vi "parseConstants.vi"(8 "error in (no error)":errorcluster, 10 "IDLString":string="module atcs {\n\tstruct LoopTime_ms {\n\t  string<32>\tprivate_revCode; //private\n\t  double\tprivate_sndStamp; //private\n\t  double\tprivate_rcvStamp; //private\n\t  long\t\tprivate_seqNum; //private\n\t  long\t\tprivate_origin; //private\n\t  long\t\tprivate_host; //private\n\t  double\tloopTime_ms;\n\t};\n\t#pragma keylist LoopTime_ms\n\tstruct Timestamp {\n\t  string<32>\tprivate_revCode; //private\n\t  double\tprivate_sndStamp; //private\n\t  double\tprivate_rcvStamp; //private\n\t  long\t\tprivate_seqNum; //private\n\t  long\t\tprivate_origin; //private\n\t  long\t\tprivate_host; //private\n\t  double\ttimestamp;\n\t};\n\t#pragma keylist Timestamp\n\tstruct command_Offset {\n\t  string<32>\tprivate_revCode; //private\n\t  double\tprivate_sndStamp; //private\n\t  double\tprivate_rcvStamp; //private\n\t  long\t\tprivate_seqNum; //private\n\t  long\t\tprivate_origin; //private\n\t  long\t\tprivate_host; //private\n\t  string<32>\tdevice;\n\t  string<32>\tproperty;\n\t  string<32>\taction;\n\t  string<32>\tvalue;\n\t  double\toffsetX;\n\t  double\toffsetY;\n\t};\n\t#pragma keylist command_Offset\n\tstruct command_SpectrographSetup {\n\t  string<32>\tprivate_revCode; //private\n\t  double\tprivate_sndStamp; //private\n\t  double\tprivate_rcvStamp; //private\n\t  long\t\tprivate_seqNum; //private\n\t  long\t\tprivate_origin; //private\n\t  long\t\tprivate_host; //private\n\t  string<32>\tdevice;\n\t  string<32>\tproperty;\n\t  string<32>\taction;\n\t  string<32>\tvalue;\n\t  long\tgrating;\n\t  long\tfilter;\n\t  double\tstagePosition;\n\t};\n\t#pragma keylist command_SpectrographSetup\n\tstruct command_Target {\n\t  string<32>\tprivate_revCode; //private\n\t  double\tprivate_sndStamp; //private\n\t  double\tprivate_rcvStamp; //private\n\t  long\t\tprivate_seqNum; //private\n\t  long\t\tprivate_origin; //private\n\t  long\t\tprivate_host; //private\n\t  string<32>\tdevice;\n\t  string<32>\tproperty;\n\t  string<32>\taction;\n\t  string<32>\tvalue;\n\t  long\ttargetId;\n\t  double\tra;\n\t  double\tdecl;\n\t  double\tskyPositionAngle;\n\t  long\tnumOfExposures;\n\t  double\texposureTime;\n\t};\n\t#pragma keylist command_Target\n\tstruct command_disable {\n\t  string<32>\tprivate_revCode; //private\n\t  double\tprivate_sndStamp; //private\n\t  double\tprivate_rcvStamp; //private\n\t  long\t\tprivate_seqNum; //private\n\t  long\t\tprivate_origin; //private\n\t  long\t\tprivate_host; //private\n\t  string<32>\tdevice;\n\t  string<32>\tproperty;\n\t  string<32>\taction;\n\t  string<32>\tvalue;\n\t  boolean\tdisable;\n\t};\n\t#pragma keylist command_disable\n\tstruct command_enable {\n\t  string<32>\tprivate_revCode; //private\n\t  double\tprivate_sndStamp; //private\n\t  double\tprivate_rcvStamp; //private\n\t  long\t\tprivate_seqNum; //private\n\t  long\t\tprivate_origin; //private\n\t  long\t\tprivate_host; //private\n\t  string<32>\tdevice;\n\t  string<32>\tproperty;\n\t  string<32>\taction;\n\t  string<32>\tvalue;\n\t  boolean\tenable;\n\t};\n\t#pragma keylist command_enable\n\tstruct command_enterControl {\n\t  string<32>\tprivate_revCode; //private\n\t  double\tprivate_sndStamp; //private\n\t  double\tprivate_rcvStamp; //private\n\t  long\t\tprivate_seqNum; //private\n\t  long\t\tprivate_origin; //private\n\t  long\t\tprivate_host; //private\n\t  string<32>\tdevice;\n\t  string<32>\tproperty;\n\t  string<32>\taction;\n\t  string<32>\tvalue;\n\t  boolean\tenterControl;\n\t};\n\t#pragma keylist command_enterControl\n\tstruct command_exitControl {\n\t  string<32>\tprivate_revCode; //private\n\t  double\tprivate_sndStamp; //private\n\t  double\tprivate_rcvStamp; //private\n\t  long\t\tprivate_seqNum; //private\n\t  long\t\tprivate_origin; //private\n\t  long\t\tprivate_host; //private\n\t  string<32>\tdevice;\n\t  string<32>\tproperty;\n\t  string<32>\taction;\n\t  string<32>\tvalue;\n\t  boolean\texitControl;\n\t};\n\t#pragma keylist command_exitControl\n\tstruct command_standby {\n\t  string<32>\tprivate_revCode; //private\n\t  double\tprivate_sndStamp; //private\n\t  double\tprivate_rcvStamp; //private\n\t  long\t\tprivate_seqNum; //private\n\t  long\t\tprivate_origin; //private\n\t  long\t\tprivate_host; //private\n\t  string<32>\tdevice;\n\t  string<32>\tproperty;\n\t  string<32>\taction;\n\t  string<32>\tvalue;\n\t  boolean\tstandBy;\n\t};\n\t#pragma keylist command_standby\n\tstruct command_start {\n\t  string<32>\tprivate_revCode; //private\n\t  double\tprivate_sndStamp; //private\n\t  double\tprivate_rcvStamp; //private\n\t  long\t\tprivate_seqNum; //private\n\t  long\t\tprivate_origin; //private\n\t  long\t\tprivate_host; //private\n\t  string<32>\tdevice;\n\t  string<32>\tproperty;\n\t  string<32>\taction;\n\t  string<32>\tvalue;\n\t  string<256>\tsettingsToApply;\n\t};\n\t#pragma keylist command_start\n\tstruct logevent_AppliedSettingsMatchStart {\n\t  string<32>\tprivate_revCode; //private\n\t  double\tprivate_sndStamp; //private\n\t  double\tprivate_rcvStamp; //private\n\t  long\t\tprivate_seqNum; //private\n\t  long\t\tprivate_origin; //private\n\t  long\t\tprivate_host; //private\n\t  boolean\tappliedSettingsMatchStartIsTrue;\n\t  long\tpriority;\n\t};\n\t#pragma keylist logevent_AppliedSettingsMatchStart\n\t\tconst long atcs_shared_SummaryState_DisabledState=1;\n\t\tconst long atcs_shared_SummaryState_EnabledState=2;\n\t\tconst long atcs_shared_SummaryState_FaultState=3;\n\t\tconst long atcs_shared_SummaryState_OfflineState=4;\n\t\tconst long atcs_shared_SummaryState_StandbyState=5;\n\t\tconst long atcs_shared_DetailedState_DisabledState=1;\n\t\tconst long atcs_shared_DetailedState_EnabledState=2;\n\t\tconst long atcs_shared_DetailedState_FaultState=3;\n\t\tconst long atcs_shared_DetailedState_OfflineState=4;\n\t\tconst long atcs_shared_DetailedState_StandbyState=5;\n\t\tconst long atcs_shared_Filter_Filter1=1;\n\t\tconst long atcs_shared_Filter_Filter2=2;\n\t\tconst long atcs_shared_Filter_Filter3=3;\n\t\tconst long atcs_shared_Filter_Filter4=4;\n\t\tconst long atcs_shared_Grating_Grating1=1;\n\t\tconst long atcs_shared_Grating_Grating2=2;\n\t\tconst long atcs_shared_Grating_Grating3=3;\n\t\tconst long atcs_shared_Grating_Grating4=4;\n\tstruct logevent_DetailedState {\n\t  string<32>\tprivate_revCode; //private\n\t  double\tprivate_sndStamp; //private\n\t  double\tprivate_rcvStamp; //private\n\t  long\t\tprivate_seqNum; //private\n\t  long\t\tprivate_origin; //private\n\t  long\t\tprivate_host; //private\n\t  long\tdetailedState;\n\t  long\tpriority;\n\t};\n\t#pragma keylist logevent_DetailedState\n\tstruct logevent_ErrorCode {\n\t  string<32>\tprivate_revCode; //private\n\t  double\tprivate_sndStamp; //private\n\t  double\tprivate_rcvStamp; //private\n\t  long\t\tprivate_seqNum; //private\n\t  long\t\tprivate_origin; //private\n\t  long\t\tprivate_host; //private\n\t  long\terrorCode;\n\t  long\tpriority;\n\t};\n\t#pragma keylist logevent_ErrorCode\n\tstruct logevent_Heartbeat {\n\t  string<32>\tprivate_revCode; //private\n\t  double\tprivate_sndStamp; //private\n\t  double\tprivate_rcvStamp; //private\n\t  long\t\tprivate_seqNum; //private\n\t  long\t\tprivate_origin; //private\n\t  long\t\tprivate_host; //private\n\t  boolean\theartbeat;\n\t  long\tpriority;\n\t};\n\t#pragma keylist logevent_Heartbeat\n\tstruct logevent_InternalCommand {\n\t  string<32>\tprivate_revCode; //private\n\t  double\tprivate_sndStamp; //private\n\t  double\tprivate_rcvStamp; //private\n\t  long\t\tprivate_seqNum; //private\n\t  long\t\tprivate_origin; //private\n\t  long\t\tprivate_host; //private\n\t  octet\tCommandObject[1000];\n\t  long\tpriority;\n\t};\n\t#pragma keylist logevent_InternalCommand\n\tstruct logevent_LoopTimeOutOfRange {\n\t  string<32>\tprivate_revCode; //private\n\t  double\tprivate_sndStamp; //private\n\t  double\tprivate_rcvStamp; //private\n\t  long\t\tprivate_seqNum; //private\n\t  long\t\tprivate_origin; //private\n\t  long\t\tprivate_host; //private\n\t  boolean\tloopTimeOutOfRange;\n\t  long\tpriority;\n\t};\n\t#pragma keylist logevent_LoopTimeOutOfRange\n\tstruct logevent_RejectedCommand {\n\t  string<32>\tprivate_revCode; //private\n\t  double\tprivate_sndStamp; //private\n\t  double\tprivate_rcvStamp; //private\n\t  long\t\tprivate_seqNum; //private\n\t  long\t\tprivate_origin; //private\n\t  long\t\tprivate_host; //private\n\t  short\tcommandValue;\n\t  long\tdetailedState;\n\t  double\ttimestamp;\n\t  long\tpriority;\n\t};\n\t#pragma keylist logevent_RejectedCommand\n\tstruct logevent_SettingVersions {\n\t  string<32>\tprivate_revCode; //private\n\t  double\tprivate_sndStamp; //private\n\t  double\tprivate_rcvStamp; //private\n\t  long\t\tprivate_seqNum; //private\n\t  long\t\tprivate_origin; //private\n\t  long\t\tprivate_host; //private\n\t  string<256>\trecommendedSettingsVersion;\n\t  string<256>\trecommendedSettingsLabels;\n\t  long\tpriority;\n\t};\n\t#pragma keylist logevent_SettingVersions\n\tstruct logevent_SpectrographInPosition {\n\t  string<32>\tprivate_revCode; //private\n\t  double\tprivate_sndStamp; //private\n\t  double\tprivate_rcvStamp; //private\n\t  long\t\tprivate_seqNum; //private\n\t  long\t\tprivate_origin; //private\n\t  long\t\tprivate_host; //private\n\t  boolean\tinPosition;\n\t  long\tpriority;\n\t};\n\t#pragma keylist logevent_SpectrographInPosition\n\tstruct logevent_SummaryState {\n\t  string<32>\tprivate_revCode; //private\n\t  double\tprivate_sndStamp; //private\n\t  double\tprivate_rcvStamp; //private\n\t  long\t\tprivate_seqNum; //private\n\t  long\t\tprivate_origin; //private\n\t  long\t\tprivate_host; //private\n\t  long\tsummaryState;\n\t  long\tpriority;\n\t};\n\t#pragma keylist logevent_SummaryState\n\tstruct logevent_TelescopeInPosition {\n\t  string<32>\tprivate_revCode; //private\n\t  double\tprivate_sndStamp; //private\n\t  double\tprivate_rcvStamp; //private\n\t  long\t\tprivate_seqNum; //private\n\t  long\t\tprivate_origin; //private\n\t  long\t\tprivate_host; //private\n\t  boolean\tinPosition;\n\t  long\tpriority;\n\t};\n\t#pragma keylist logevent_TelescopeInPosition\n\tstruct logevent_TelescopeSkyPosition {\n\t  string<32>\tprivate_revCode; //private\n\t  double\tprivate_sndStamp; //private\n\t  double\tprivate_rcvStamp; //private\n\t  long\t\tprivate_seqNum; //private\n\t  long\t\tprivate_origin; //private\n\t  long\t\tprivate_host; //private\n\t  double\ttimestamp;\n\t  double\traTel;\n\t  double\tdecTel;\n\t  double\tskyPositionAngleTel;\n\t  long\tpriority;\n\t};\n\t#pragma keylist logevent_TelescopeSkyPosition\n\tstruct command\n\t{\n      string<32>\tprivate_revCode;\n      double\t\tprivate_sndStamp;\n      double\t\tprivate_rcvStamp;\n      long\t\tprivate_origin;\n      long \t\tprivate_host;\n      long\t\tprivate_seqNum;\n      string<32>\tdevice;\n      string<32>\tproperty;\n      string<32>\taction;\n      string<32>\tvalue;\n      string<128>\tmodifiers;\n\t};\n\t#pragma keylist command\n\tstruct ackcmd\n\t{\n      string<32>\tprivate_revCode;\n      double\t\tprivate_sndStamp;\n      double\t\tprivate_rcvStamp;\n      long\t\tprivate_origin;\n      long \t\tprivate_host;\n      long\t\tprivate_seqNum;\n      long \t\tack;\n      long \t\terror;\n      string<256>\tresult;\n\t};\n\t#pragma keylist ackcmd\n\tstruct logevent\n\t{\n      string<32>\tprivate_revCode;\n      double\t\tprivate_sndStamp;\n      double\t\tprivate_rcvStamp;\n      long\t\tprivate_origin;\n      long \t\tprivate_host;\n      string<128>\tmessage;\n\t};\n\t#pragma keylist logevent\n};\n", 11 "Enumeration in":refnum<class "Enumeration.lvclass">) -> (0 "error out":errorcluster, 2 "IDLConstants":string, 3 "Enumeration out":refnum<class "Enumeration.lvclass">)   [LabVIEW 2016, in "Enumeration.lvclass"]
uses:
  Enumeration.lvclass
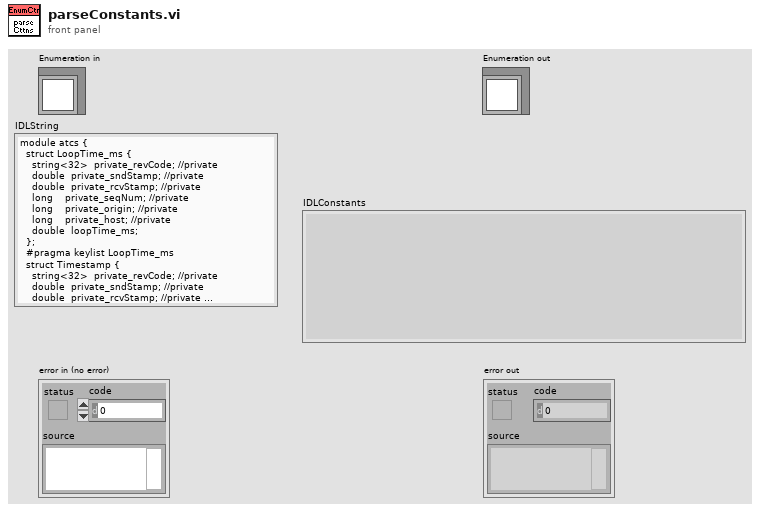
[diagram p1: front panel]
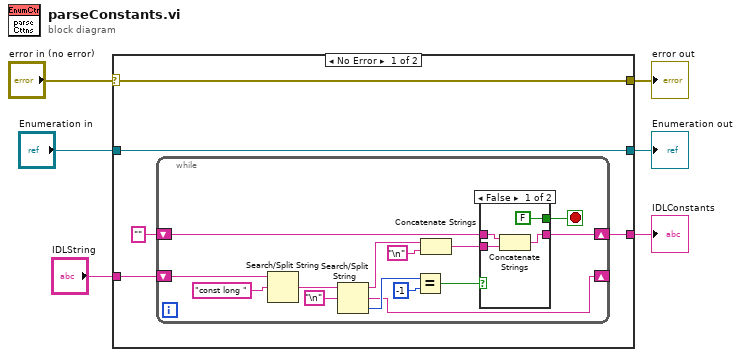
[diagram p0: block diagram]
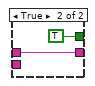
[diagram p2: hidden frame]
diagram:
  n1 = case shown="No Error" "error in (no error)" {
    selector: "error in (no error)" -> [w11 w33]
    tunnel: [w11 w33] -> w5
    tunnel: [w8 w32] -> w3
    tunnel: "Enumeration in" -> [w8 w32]
    tunnel: "IDLString" -> [w9 _]
    tunnel: [w7 _] -> w1
    frame No Error {
      n2 = while {
        shift-right: [w17] -> w7
        shift-left: "" -> [w18]
        shift-right: [w13] -> _
        shift-left: w9 -> [w24]
        stop <- w19 stop-if-true
        n3 = Search/Split String(string=w24, search string/char (-)="const long ") -> (match + rest of string=w23:string)  [unwired: 1 in, 2 out]
        n4 = Search/Split String(string=w23, search string/char (-)="\n") -> (substring before match=w16:string, match + rest of string=w13:string, offset of match=w21:i32)  [unwired: 1 in]
        n5 = Equal?(x=w21, y=-1) -> (x = y?=w20:bool)
        n6 = Concatenate Strings(w16, "\n") -> (w14:string)
        n7 = case shown="False" w20 {
          tunnel: [FALSE TRUE] -> w19
          tunnel: w18 -> [w28 w30]
          tunnel: [w27 w30] -> w17
          tunnel: w14 -> [w26 _]
          frame False {
            n8 = Concatenate Strings(w28, w26) -> (w27:string)
          }
          frame True {
          }
        }
      }
    }
    frame Error {
    }
  }
  "error out" <- w5
  "Enumeration out" <- w3
  "IDLConstants" <- w1
